vi "RM.checkReservation.vi"(5 "Resource Type":T1, 7 "Direction":T2, 8 "error in":errorcluster, 10 "name in bitfile":string, 11 "reservation DB in":variant) -> (0 "error out":errorcluster, 1 "clientGUID":string, 2 "found?":bool, 3 "reservation DB out":variant)   [LabVIEW 2016, in "FPGA Resource Manager.lvlib"]
uses:
  FPGA Resource Manager.lvlib
  RM.resourceDirection.ctl
  RM.resourceType.ctl
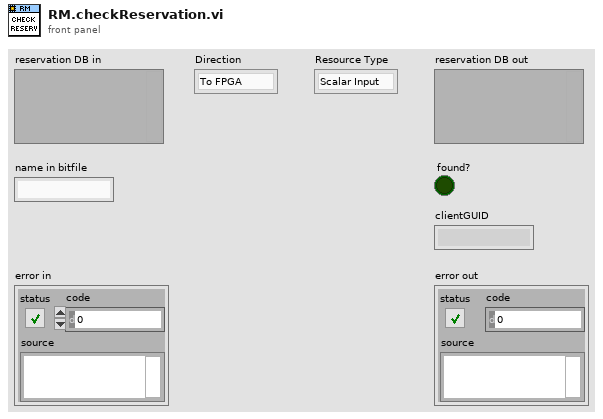
[diagram p1: front panel]
types:
  T1 = typedef "FPGA Resource Manager.lvlib/RM.resourceType.ctl" = enum16{"Scalar Input", "Scalar Output", "Waveform Input", "Waveform Output"}
  T2 = typedef "FPGA Resource Manager.lvlib/RM.resourceDirection.ctl" = enum16{"To FPGA", "From FPGA"}
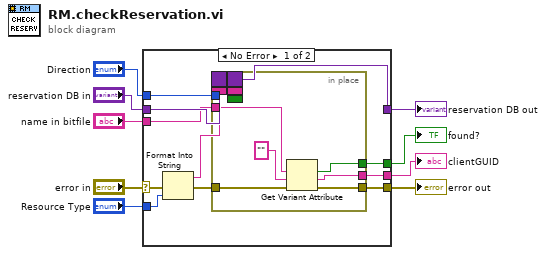
[diagram p0: block diagram]
diagram:
  n1 = case shown="No Error" "error in" {
    selector: "error in" -> [w13 w29]
    tunnel: "reservation DB in" -> [w20 w30]
    tunnel: "Direction" -> [w19 _]
    tunnel: [w18 w30] -> w2
    tunnel: "name in bitfile" -> [w17 _]
    tunnel: "Resource Type" -> [w16 _]
    tunnel: [w12 w29] -> w4
    tunnel: [w11 _] -> w3
    tunnel: [w10 _] -> w1
    frame No Error {
      n2 = Format Into String(error in=w13, w16) -> (resulting string=w15:string, error out=w14:errorcluster)  [unwired: 2 in]
      n3 = in-place {
        in-place-border: w19 -> [_]
        in-place-border: w17 -> [w28]
        in-place-border: w14 -> [w27]
        in-place-border: [w26] -> w12
        in-place-border: [w25] -> w11
        border: w20 -> [_]
        border: w15 -> [_]
        border: [_] -> w18
        border: _ -> [_]
        border: _ -> [_]
        in-place-border: [w24] -> w10
        n4 = Get Variant Attribute(Variant=w22, name=w28, default value (empty Variant)="" ("name in bitfile"), error in=w27) -> (duplicate Variant=w21:variant, found=w25:bool, value=w24:string, error out=w26:errorcluster)
      }
    }
    frame Error {
    }
  }
  "reservation DB out" <- w2
  "error out" <- w4
  "found?" <- w3
  "clientGUID" <- w1
